vi "handle-select-frame.vi"(4 "symbol":i32, 6 "Indent Level":i32, 8 "error in (no error)":errorcluster, 9 "open?":bool, 10 "Tag":string, 11 "dbc in":refnum<class "dbc.lvclass">) -> (0 "error out":errorcluster, 1 "frame.def":T1={"CAN.frame"={"Comment"="", "Extended Identifier?"=FALSE, "Transmit Time"=0.0, "Timing Type"=1, "Payload Length"=8, "Identifier"=1, "Frame name"="frame1"}, "frame.type"=enum."FRAME NOT DEFINED"} {"CAN.frame"."Timing Type" items=["Cyclic Data", "Event Data", "Cyclic Remote", "Event Remote"]; "CAN.frame"."Identifier" format="%010x"}, 2 "payload":bool[][](array[boolean]), 3 "dbc out":refnum<class "dbc.lvclass">)   [LabVIEW 2015]
uses:
  dbc.lvclass
  subs/frame-defination.ctl
  controls/dbc-frame.ctl
  subs/frame.type.ctl
  dbc.lvclass/dbc.ctl
  Write-active-item-tag.vi
  Write-active-frame-tag.vi
  Write-active-item-indent-lvl.vi
  Write-active-item-symbol.vi
  class.can.table/bAPPdata.lvclass
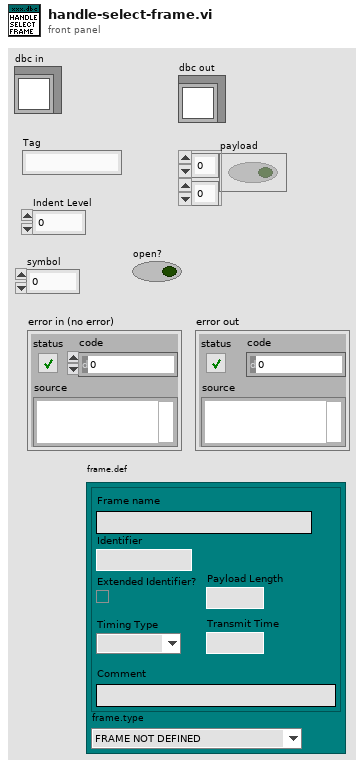
[diagram p1: front panel]
types:
  T1 = typedef "frame-defination.ctl" = cluster{"CAN.frame":T2, "frame.type":T3}
  T2 = typedef "dbc-frame.ctl" = cluster{"Comment":string, "Extended Identifier?":bool, "Transmit Time":dbl, "Timing Type":u32, "Payload Length":u32, "Identifier":u32, "Frame name":string}
  T3 = typedef "frame.type.ctl" = enum16{"FRAME NOT DEFINED", "DUT OUTPUT FRAME", "DUT INPUT FRAME"}
  T4 = typedef "XNET Frame CAN.ctl" = cluster{"timestamp":timestamp, "payload":u8[], "identifier":u32, "type":T5, "extended?":bool, "echo?":bool}
  T5 = typedef "XNET Frame Type CAN.ctl" = u8
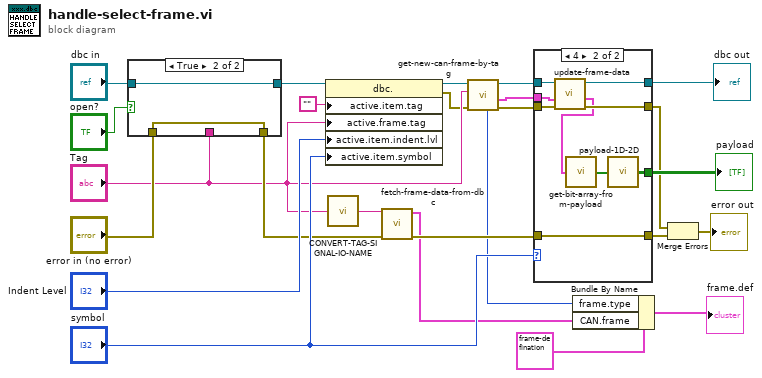
[diagram p0: block diagram]
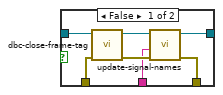
[diagram p2: hidden frame]
diagram:
  n1 = case shown="True" "open?" {
    tunnel: "error in (no error)" -> [w32 w33]
    tunnel: "dbc in" -> [w31 w34]
    tunnel: [w29 w34] -> w18
    tunnel: [w27 w33] -> w13
    tunnel: "Tag" -> [w26 _]
    frame False {
      n2 = call "dbc-close-frame-tag.vi"("error in (no error)"=w32, "dbc in"=w31) -> ("error out"=w28:errorcluster, "dbc out"=w30:refnum<class "dbc.lvclass">)  [unwired: 8 in]
      n3 = call "update-signal-names.vi"("error in (no error)"=w28, "frame.tag"=w26, "dbc in"=w30) -> ("error out"=w27:errorcluster, "dbc out"=w29:refnum<class "dbc.lvclass">)  [unwired: 7 in]
    }
    frame True {
    }
  }
  n4 = property class="dbc."(reference=w18, "active.item.tag"="", "active.frame.tag"="Tag", "active.item.indent.lvl"="Indent Level", "active.item.symbol"="symbol") -> (reference out=w16:refnum<class "dbc.lvclass">, error out=w10:errorcluster)  [unwired: 1 in]
  n5 = call "CONVERT-TAG-SIGNAL-IO-NAME.vi"("tag"="Tag") -> ("signal"=w6:string)  [unwired: 4 in]
  n6 = call "fetch-frame-data-from-dbc.vi"("error in (no error)"=w13, "frame.tag"=w6) -> ("error out"=w7:errorcluster, "frame"=w3:T2)  [unwired: 8 in]
  n7 = call "get-new-can-frame-by-tag.vi"("error in (no error)"=w10, "tag"="Tag", "CANtable in"=w16) -> ("error out"=w9:errorcluster, "CAN frame"=w8:T4, "CANtable out"=w12:refnum<class "dbc.lvclass">, "frame.type"=w2:T3)  [unwired: 5 in]
  n8 = case shown="4" "symbol" {
    tunnel: w12 -> [w37 w41]
    tunnel: [w37 w46] -> w20
    tunnel: [w36 w43] -> w15
    tunnel: w7 -> [w36 w43]
    tunnel: w9 -> [w35 w40]
    tunnel: [w35 w45] -> w14
    tunnel: [_ w42] -> w24
    tunnel: w8 -> [_ w39]
    frame 0, Default {
    }
    frame 4 {
      n9 = call "update-frame-data.vi"("error in (no error)"=w40, "id"=w39, "dbc in"=w41) -> ("error out"=w45:errorcluster, "CAN frame"=w38:T4, "dbc out"=w46:refnum<class "dbc.lvclass">)  [unwired: 6 in]
      n10 = call "get-bit-array-from-payload.vi"("CAN frame"=w38) -> ("Array"=w44:bool[])  [unwired: 4 in]
      n11 = call "payload-1D-2D.vi"("Array"=w44) -> ("Array 2"=w42:bool[][])  [unwired: 4 in]
    }
  }
  "payload" <- w24
  "dbc out" <- w20
  n12 = Bundle By Name(cluster=T1 {"CAN.frame"={"Comment"="", "Extended Identifier?"=FALSE, "Transmit Time"=0.0, "Timing Type"=1, "Payload Length"=8, "Identifier"=1, "Frame name"="frame1"}, "frame.type"=enum."FRAME NOT DEFINED"} ("frame.def"), "frame.type"=w2, "CAN.frame"=w3) -> (→"frame.def":T1)
  n13 = Merge Errors(w14, w15) -> (→"error out":errorcluster)
